vi "Pendulum is Buffer Ready.vi"(10 "packetsWorth":i32, 11 "instance":i32) -> (3 "function return":i32)   [LabVIEW 2024, in "pendulumApp.lvlib"]
doc: "OOTB_API int Pendulum_isBufferReady(int instance,int packetsWorth);"
uses:
  pendulumApp.lvlib
  pendulumApp.dll
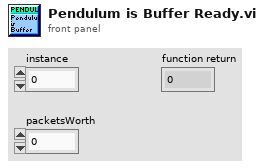
[diagram p1: front panel]
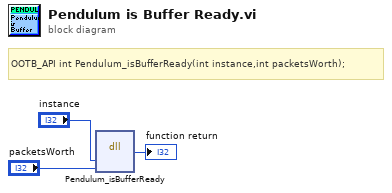
[diagram p0: block diagram]
diagram:
  # "OOTB_API\tint Pendulum_isBufferReady(int instance,int packetsWorth);"
  n1 = dll-call lib="C:/Users/scer/OneDrive - University of Florida/eml4314c/eml4314cFA25/Resources/FA25_dev_version2/SADI_Pendulum_lib/pendulumApp.*" fn="Pendulum_isBufferReady"("instance"="instance", "packetsWorth"="packetsWorth") -> (→"function return":i32)  [unwired: 5 in, 2 out]
